vi "Info Replace Scalar.vi"(7 "key description to replace":string, 10 "info data to paste":string, 11 "info data in":string) -> (3 "info data out":string)   [LabVIEW 2020]
doc: "Addition to infolib: Replaces scalar section by another string input."
uses:
  <vilib>/regexp/Match Regular Expression.xnode
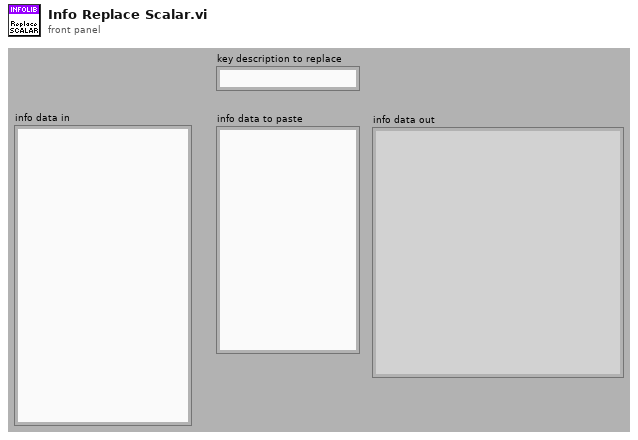
[diagram p1: front panel]
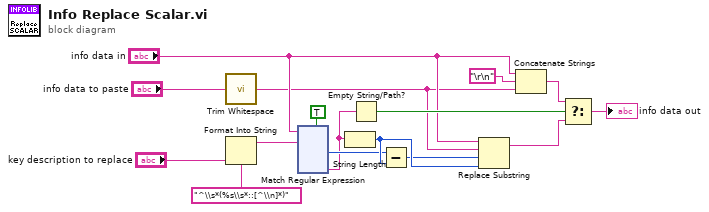
[diagram p0: block diagram]
diagram:
  n1 = call <vilib>:"Trim Whitespace.vi"("string"="info data to paste") -> ("trimmed string"=w1:string)  [unwired: 1 in]
  n2 = Format Into String(format string="^\\s*(%s\\s*::[^\\n]*)", "key description to replace") -> (resulting string=w13:string)  [unwired: 2 in, 1 out]
  n3 = xnode "Match Regular Expression"("input string"="info data in", "regular expression"=w13, "multiline? (F)"=TRUE) -> ("offset past match"=w15:i32, "submatch 1"=w8:string)  [unwired: 3 in, 4 out]
  n4 = String Length(string=w8) -> (length=w16:i32)
  n5 = Empty String/Path?(string/path=w8) -> (empty?=w7:bool)
  n6 = Subtract(x=w15, y=w16) -> (x-y=w12:i32)
  n7 = Replace Substring(2:w16, 3:w12, 4:w1, 5:"info data in") -> (1:w6:string)  [unwired: 1 out]
  n8 = Concatenate Strings("info data in", "\r\n", w1) -> (w4:string)
  n9 = Select(t=w4, s=w7, f=w6) -> (s? t:f=→"info data out":string)
